vi "DPIDs.Initialize.vi"(7 "Read Lookup":variant, 8 "error in":errorcluster, 9 "DPID Lookup":variant, 10 "UUDT Receive ID":u32=513 format="%.0x", 11 "cluster in":refnum<k21>) -> (0 "error out":errorcluster, 1 "DPID Lookup Out":variant, 2 "GMLAN DPID Session":refnum<k21>, 3 "Cluster Out":refnum<k21>)   [LabVIEW 2015, in "Diagnostics Addon Engine.lvlib"]
uses:
  Diagnostics Addon Engine.lvlib
  Shared/Types/XNET.Frame.ctl
  Shared/Types/DPID.Lookup.Info.ctl
  Shared/Types/DPID.Lookup.Info.PID.ctl
  Shared/Types/Frame.Lookup.Info.ctl
  Shared/Types/Type.ctl
  Shared/SubVIs/Constants.vi
  Shared/Diagnostics Addon Shared.lvlib
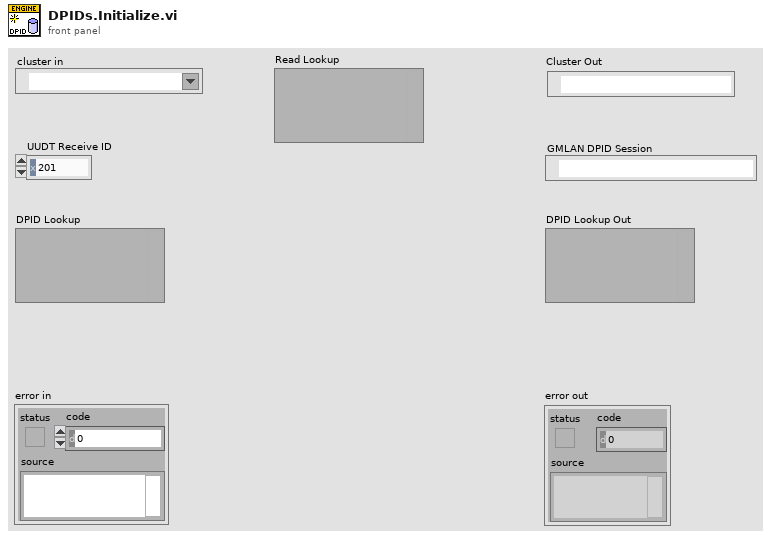
[diagram p1: front panel]
types:
  T1 = typedef "Diagnostics Addon Shared.lvlib/XNET.Frame.ctl" = cluster{"Frame name":string, "Identifier":u32, "Payload Length":u32, "Timing Type":u32, "Transmit Time":dbl, "Extended Identifier?":bool, "Comment":string}
  T2 = typedef "Diagnostics Addon Shared.lvlib/DPID.Lookup.Info.ctl" = cluster{"PID Info":T3, "Datatable Lookup":T4, "Conversion":refnum<k21>}
  T3 = typedef "Diagnostics Addon Shared.lvlib/DPID.Lookup.Info.PID.ctl" = cluster{"PID":u16, "Frame Length":u8}
  T4 = typedef "Diagnostics Addon Shared.lvlib/Frame.Lookup.Info.ctl" = cluster{"Offset":i32, "Length":i32, "ByteLength":u16}
  T5 = typedef "Diagnostics Addon Shared.lvlib/Type.ctl" = enum16{"DID", "CDID", "PID", "CPID", "Read Memory", "Write Memory", "DTC Control", "IO Cmd", "IO Resp", "Routine Start Cmd", "Routine Start Resp", "Routine Request Cmd", "Routine Request Resp", "Routine Stop Cmd", "Routine Stop Resp", "UserDefined Cmd", "UserDefined Rsp"}
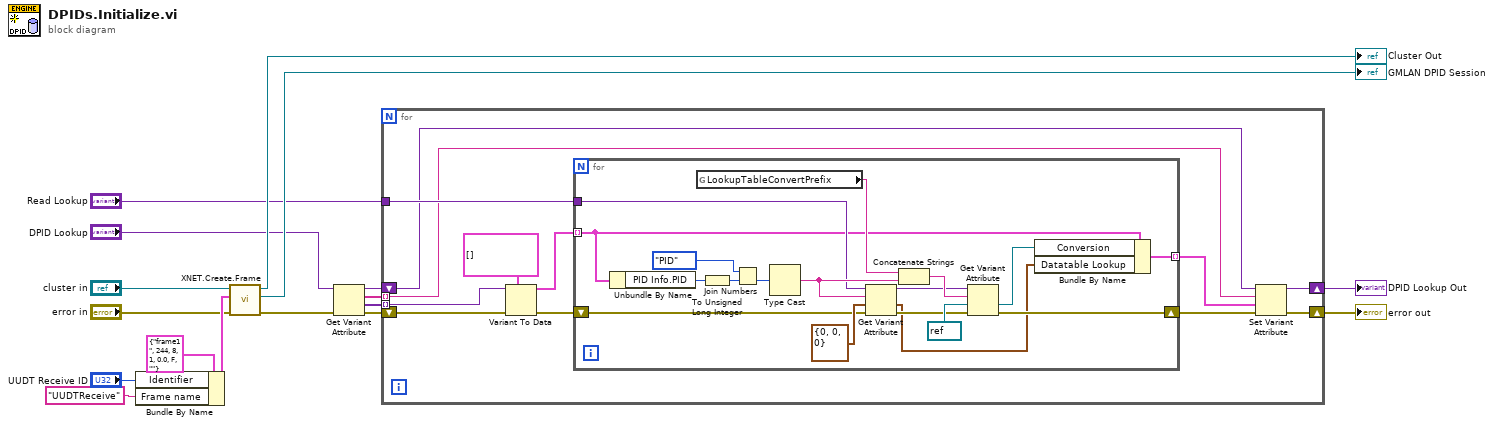
[diagram p0: block diagram]
diagram:
  n1 = Bundle By Name(cluster=T1 {"Frame name"="frame1", "Identifier"=244, "Payload Length"=8, "Timing Type"=1, "Transmit Time"=0.0, "Extended Identifier?"=FALSE, "Comment"=""} ("CAN Frame"), "Identifier"="UUDT Receive ID", "Frame name"="UUDTReceive") -> (w15:T1)
  n2 = call "XNET.Create.Frame.vi"("error in"="error in", "CAN Frame"=w15, "cluster in"="cluster in") -> ("error out"=w2:errorcluster, "frame out"=→"GMLAN DPID Session":refnum<k21>, "cluster out"=→"Cluster Out":refnum<k21>)  [unwired: 6 in]
  n3 = Get Variant Attribute(Variant="DPID Lookup", error in=w2) -> (duplicate Variant=w4:variant, names=w5:string[], values=w8:variant[], error out=w7:errorcluster)  [unwired: 2 in]
  n4 = for {
    tunnel: w8 -> [w28] mode=indexing
    tunnel: "Read Lookup" -> [w24]
    tunnel: w5 -> [w18] mode=indexing
    shift-right: [w19] -> w3
    shift-left: w4 -> [w20]
    shift-right: [w22] -> w1
    shift-left: w7 -> [w29]
    n5 = Variant To Data(error in=w29, type=T2[] [], Variant=w28) -> (data=w26:T2[], error out=w25:errorcluster)
    n6 = for {
      tunnel: w26 -> [w33] mode=indexing
      shift-right: [w38] -> w23
      shift-left: w25 -> [w42]
      tunnel: w24 -> [w40]
      tunnel: [w34] -> w21 mode=indexing
      n7 = Unbundle By Name(w33) -> ("PID Info.PID"=w35:u16)
      n8 = global read "Constants.vi" "LookupTableConvertPrefix"() -> (w45:string)
      n9 = To Unsigned Long Integer(number=w35) -> (unsigned 32bit integer=w32:u32)
      n10 = Join Numbers(hi=Type."PID" ("DID/PID"), lo=w32) -> ((hi.lo)=w31:u64)
      n11 = Type Cast(x=w31) -> (*(type *) &x=w41:string)  [unwired: 1 in]
      n12 = Get Variant Attribute(Variant=w40, name=w41, default value (empty Variant)=T4 {"Offset"=0, "Length"=0, "ByteLength"=0} ("cluster"), error in=w42) -> (duplicate Variant=w39:variant, value=w36:T4, error out=w43:errorcluster)  [unwired: 1 out]
      n13 = Concatenate Strings(w45, w41) -> (w46:string)
      n14 = Get Variant Attribute(Variant=w39, name=w46, default value (empty Variant)=refnum<k21> refnum ("DID Conversion"), error in=w43) -> (value=w37:refnum<k21>, error out=w38:errorcluster)  [unwired: 2 out]
      n15 = Bundle By Name(cluster=w33, "Conversion"=w37, "Datatable Lookup"=w36) -> (w34:T2)
    }
    n16 = Set Variant Attribute(Variant=w20, name=w18, value=w21, error in=w23) -> (Variant out=w19:variant, error out=w22:errorcluster)  [unwired: 1 out]
  }
  "error out" <- w1
  "DPID Lookup Out" <- w3
